vi "Set Cell Data.vi"(8 "error in (no error)":errorcluster, 10 "Cell Data":string[][](array[string]), 11 "MCListbox with Checkboxes in":refnum<class "MCListbox with Checkboxes.lvclass">) -> (0 "error out":errorcluster, 3 "MCListbox with Checkboxes out":refnum<class "MCListbox with Checkboxes.lvclass">)   [LabVIEW 2016, in "MCListbox with Checkboxes.lvclass"]
uses:
  MCListbox with Checkboxes.lvclass
  MCListbox with Checkboxes.lvclass/MCListbox with Checkboxes.ctl
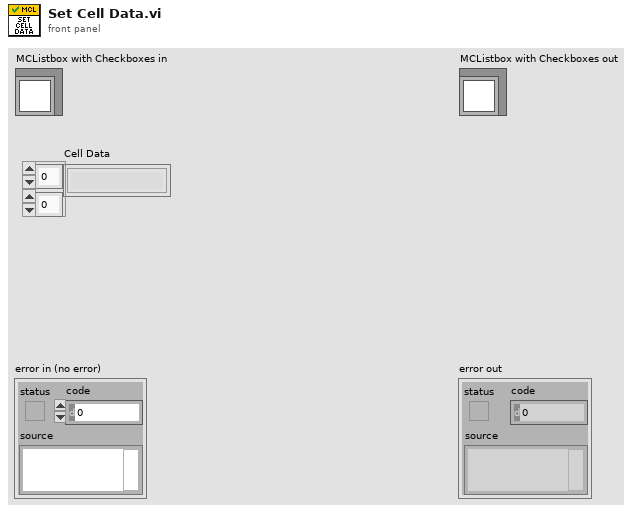
[diagram p1: front panel]
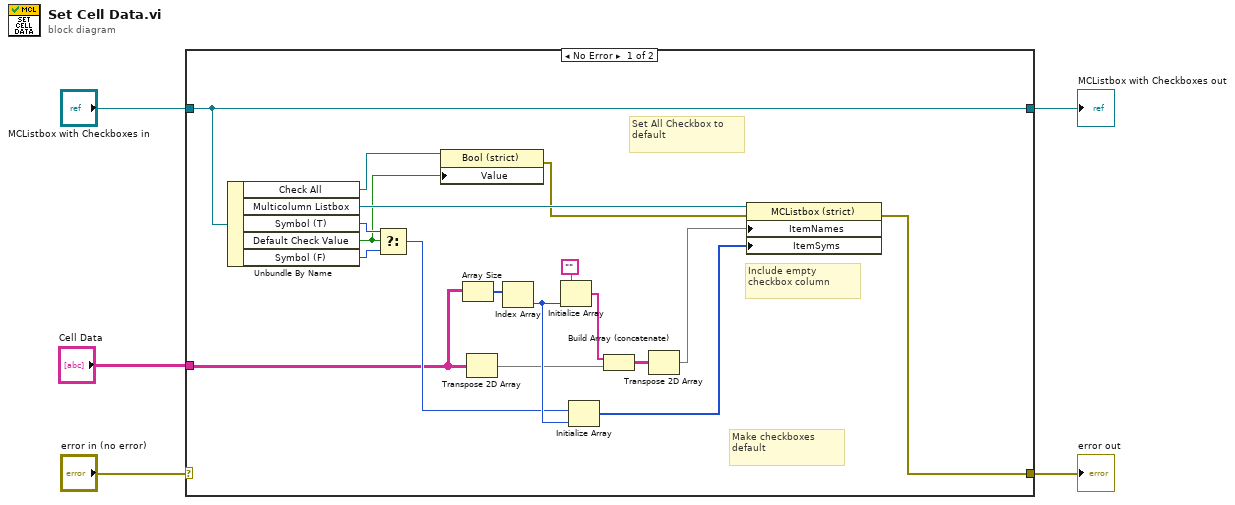
[diagram p0: block diagram]
diagram:
  n1 = case shown="No Error" "error in (no error)" {
    selector: "error in (no error)" -> [_ w25]
    tunnel: [w11 w25] -> w4
    tunnel: [w23 w24] -> w2
    tunnel: "MCListbox with Checkboxes in" -> [w23 w24]
    tunnel: "Cell Data" -> [w10 _]
    frame No Error {
      # "Set All Checkbox to default"
      # "Make checkboxes default"
      # "Include empty checkbox column"
      n2 = Unbundle By Name(w23) -> ("Check All"=w14:refnum<vi>, "Multicolumn Listbox"=w22:refnum<vi>, "Symbol (T)"=w17:i32, "Default Check Value"=w13:bool, "Symbol (F)"=w16:i32)
      n3 = Select(t=w17, s=w13, f=w16) -> (s? t:f=w15:i32)
      n4 = property class="Bool (strict)"(reference=w14, "Value"=w13) -> (error out=w12:errorcluster)  [unwired: 1 in, 1 out]
      n5 = Array Size(array=w10) -> (size(s)=w21:i32[])
      n6 = Transpose 2D Array(2D array=w10) -> (transposed array=w8:string[][])
      n7 = Index Array(array=w21) -> (element=w19:i32)  [unwired: 1 in]
      n8 = Initialize Array("", w19) -> (w9:string[])
      n9 = Initialize Array(w15, w19) -> (w18:i32[])
      n10 = Build Array (concatenate)(w9, w8) -> (w7:string[][])
      n11 = Transpose 2D Array(2D array=w7) -> (transposed array=w6:string[][])
      n12 = property class="MCListbox (strict)"(reference=w22, error in=w12, "ItemNames"=w6, "ItemSyms"=w18) -> (error out=w11:errorcluster)  [unwired: 1 out]
    }
    frame Error {
    }
  }
  "error out" <- w4
  "MCListbox with Checkboxes out" <- w2
